vi "Aux CO2 Serial Write and Read.vi"(4 "error in":errorcluster, 5 "Action":T2, 6 "string to write":string, 7 "Serial Port":T1={"termination char"=10, "End read on termination character?"=TRUE, "Enabled?"=FALSE, "VISA resource name"="COM7", "baud rate"=9600, "data bits"=8, "parity"=enum."None", "stop bits"=10, "flow control"=0, "timeout (ms)"=10000, "Input buffer size"=4096, "End write on termination character?"=FALSE, "XON Char"=17, "XOFF Char"=19} {"XOFF Char" format="%.0x"; "XON Char" format="%.0x"; "flow control" items=["None"=0, "XON/XOFF"=1, "RTS/CTS"=2, "DTR/DSR"=4]; "stop bits" items=["1.0"=10, "1.5"=15, "2.0"=20]; "baud rate" items=["1.0"=10, "1.5"=15, "2.0"=20]; "termination char" format="%.0x"}) -> (0 "error IO":errorcluster, 1 "bytes read":i16=5, 2 "read string":string="\n", 3 "Serial Port Out":T1={"termination char"=10, "End read on termination character?"=TRUE, "Enabled?"=TRUE, "VISA resource name"="COM1", "baud rate"=9600, "data bits"=8, "parity"=enum."None", "stop bits"=10, "flow control"=0, "timeout (ms)"=10000, "Input buffer size"=4096, "End write on termination character?"=FALSE, "XON Char"=17, "XOFF Char"=19} {"XOFF Char" format="%.0x"; "XON Char" format="%.0x"; "flow control" items=["None"=0, "XON/XOFF"=1, "RTS/CTS"=2, "DTR/DSR"=4]; "stop bits" items=["1.0"=10, "1.5"=15, "2.0"=20]; "baud rate" items=["1.0"=10, "1.5"=15, "2.0"=20]; "termination char" format="%.0x"})   [LabVIEW 2016]
doc: "The Advanced Serial Read and Write example performs a Serial Port Read, a Serial Port Write, or a combination of these actions while setting some advanced serial features like buffer size, termination characters, and XON/XOFF flow control. The user selects the actions (read or write) on the front panel. If both are selected, the VI will write the data first, read the data and then close the VISA session that is opened to the port. \n\nThe parameters set for the serial port must match the parameters of the connected instrument or device. In this example, the bytes to read parameter specifies the number of bytes that the serial port reads. If there were more bytes at the port than the number specified in bytes to read, those bytes would not be read. Also, if you specify to read more bytes than the number of bytes actually read, you might receive a timeout error message.\n\nINSTRUCTIONS:\n1) Select the serial resource and configuration parameters (baud rate, data bits, parity, stop bits, flow control).\n2) Termination character can be enabled and set. Also, set the required input buffer size prior to running the example.\n3) Select the operations to be performed. \n4) Connect the serial port to your device. If no device is available, perform a loopback test by doing one of the following. Short pins 2 and 3 on a RS-232 cable or short pin 4 to pin 8 and pin 5 to pin 9 on a RS-485/422 cable. \n5) Run the VI to see the data read. (The \"read string\" will match the \"string to write\" if a loopback test was performed.)\n\nThis example exposes several advanced features that you may need for your application. Not all applications need all the features shown in this example. The input buffer size is likely an important setting that you want to control in your application. This example expands upon the flow control option for XON and XOFF, allowing the user to choose those control characters. The timeout parameter has been brought to the front panel so a user can specify the time period the VISA Read will wait for the number of bytes to read before timing out. Also, the user has several controls for the termination character, which is discussed later.\n\nNote that you can press the write and read buttons and change the bytes to read parameters on the fly, while the example is running. However, you must stop the example to change the other configuration parameters after the example has started running, and then run again.\n\nSet the I/O buffer size slightly higher the amount of data you expect to receive. This is very important for applications that don't use flow control, as you may lose characters if the receive buffer overflows.\n\nSetting the timeout period ensures that the operation returns with a timeout error if the operation cannot be performed in the specified time period. \n\nSome devices require a termination character in order to identify the end of command strings. Some devices send a termination character to signify the end of data to be read. \n\nThis example shows how you can end the Read operation once a termination character is detected in the buffer and/or append a termination character at the end of the Write data. To enable the Read to end on a termination character, use the VISA Configure Serial Port or use the VISA Properties Serial End Mode for Reads, Termination Character Enable, and Termination Character. To end the Write with a termination character, use the VISA Properties Serial End Mode for Writes, the Send End Enable, and Termination Character. In this example, the same termination character is used for both the Read and the Write. You can specify two different characters for your application, if desired.\n\nYour application may require specific characters for the XON/XOFF Flow Control. You can specify these characters with the VISA Properties Flow Control XOFF Character and Flow Control XON Character. Note that if the standard XON and XOFF characters are used, then decimal 17 and 19 are unavailable for data values. Remember that using flow control and setting an adequate buffer size allow you to prevent buffer overflows."
uses:
  Controls/Serial Visa Control.ctl
  Controls/SerialPortControl.ctl
  <vilib>/Instr/_visa.llb/VISA Configure Serial Port (Instr).vi
panel:
  # "Select the serial resource and the operations to be performed.  If all are selected, the VI will write the data first, read data and then close the VISA session that is opened to the port.  This VI will wait until the specified number of bytes is received at the port until the timeout period is met.  Only the specified number of bytes will be read unless the read ends on a termination character.  The termination character can be enabled and set.  Also, set the required input buffer size prior to running the example.\nNote: The example loops until the STOP button is pressed."
  # "For additional information select File >> VI Properties >> Documentation"
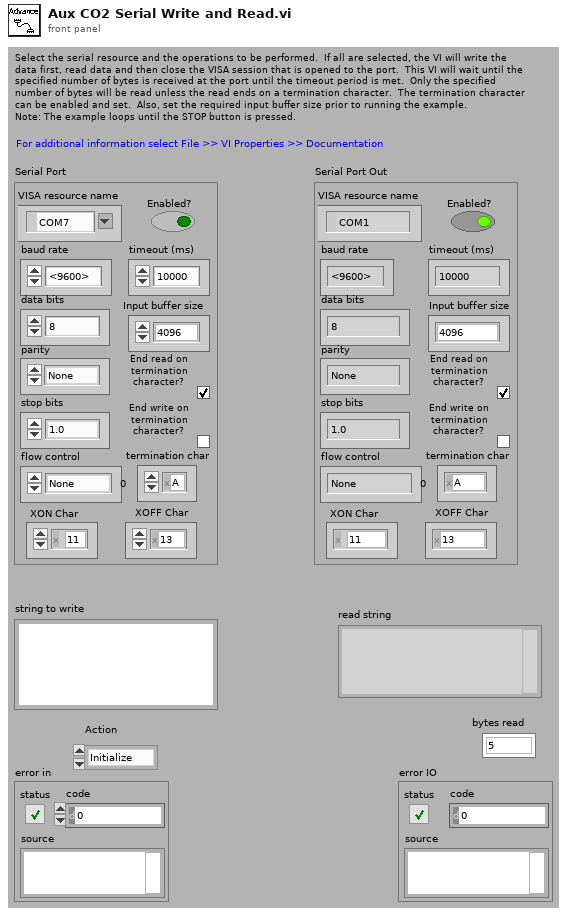
[diagram p1: front panel]
types:
  T1 = typedef "Serial Visa Control.ctl" = cluster{"termination char":u8, "End read on termination character?":bool, "Enabled?":bool, "VISA resource name":refnum<visa-resource-name>, "baud rate":u32, "data bits":u16, "parity":enum16{"None", "Odd", "Even", "Mark", "Space"}, "stop bits":u16, "flow control":u16, "timeout (ms)":u32, "Input buffer size":u32, "End write on termination character?":bool, "XON Char":u8, "XOFF Char":u8}
  T2 = typedef "SerialPortControl.ctl" = enum16{"Initialize", "Write Data", "Read Data", "Close Port"}
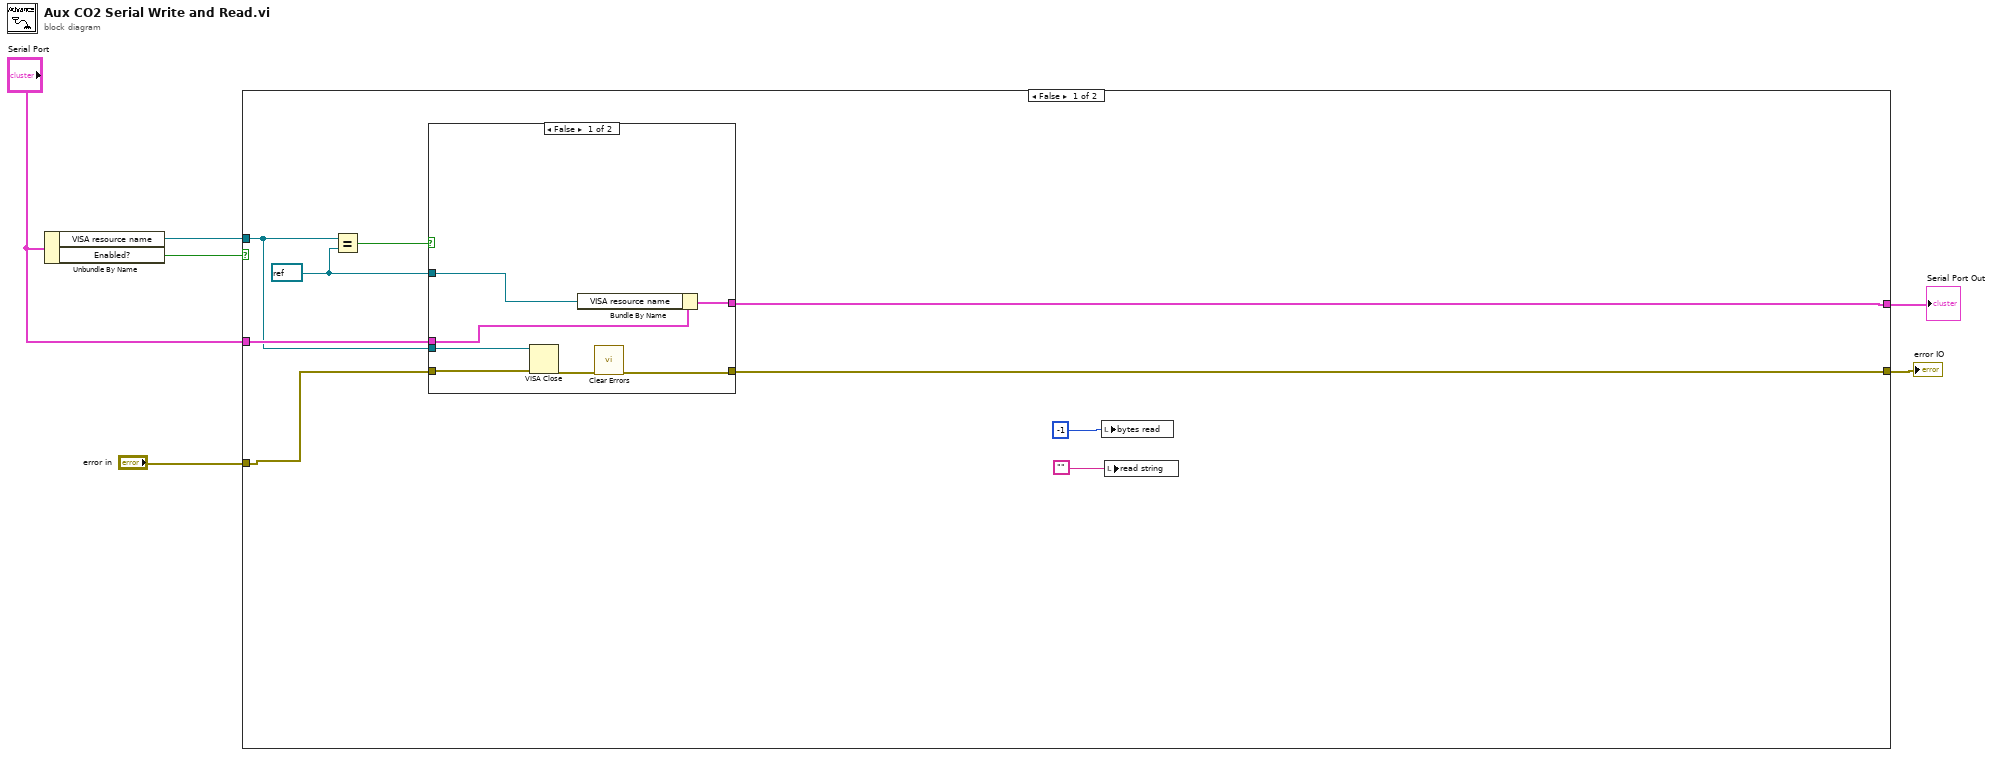
[diagram p0: block diagram]
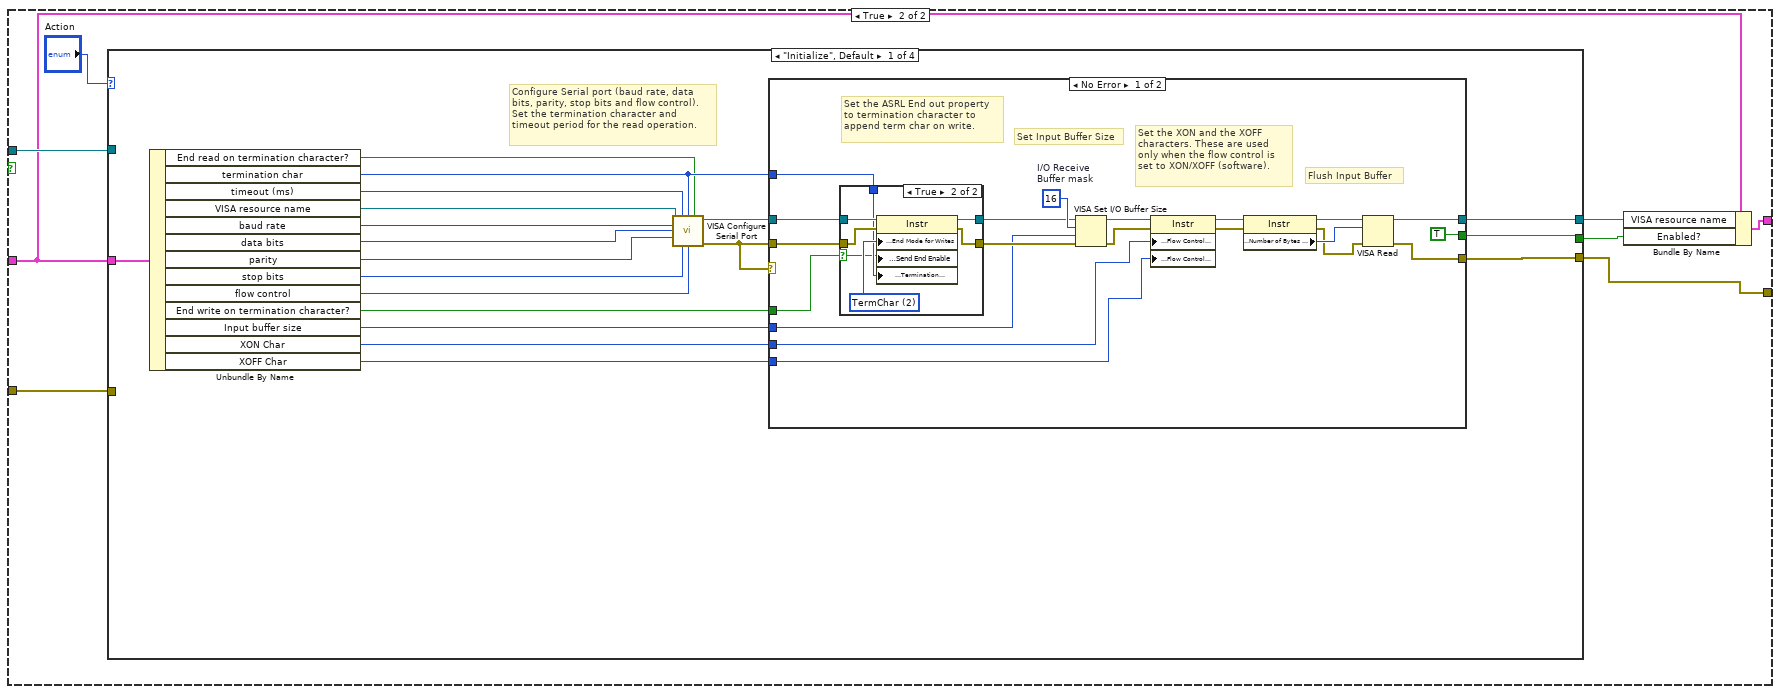
[diagram p3: hidden frame]
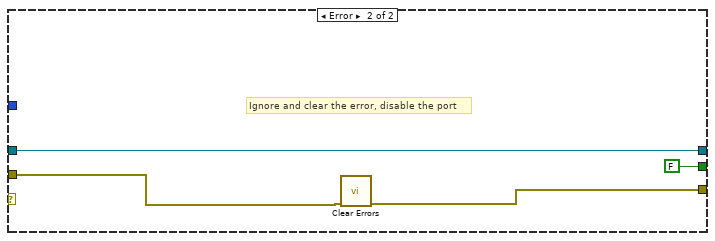
[diagram p5: hidden frame]
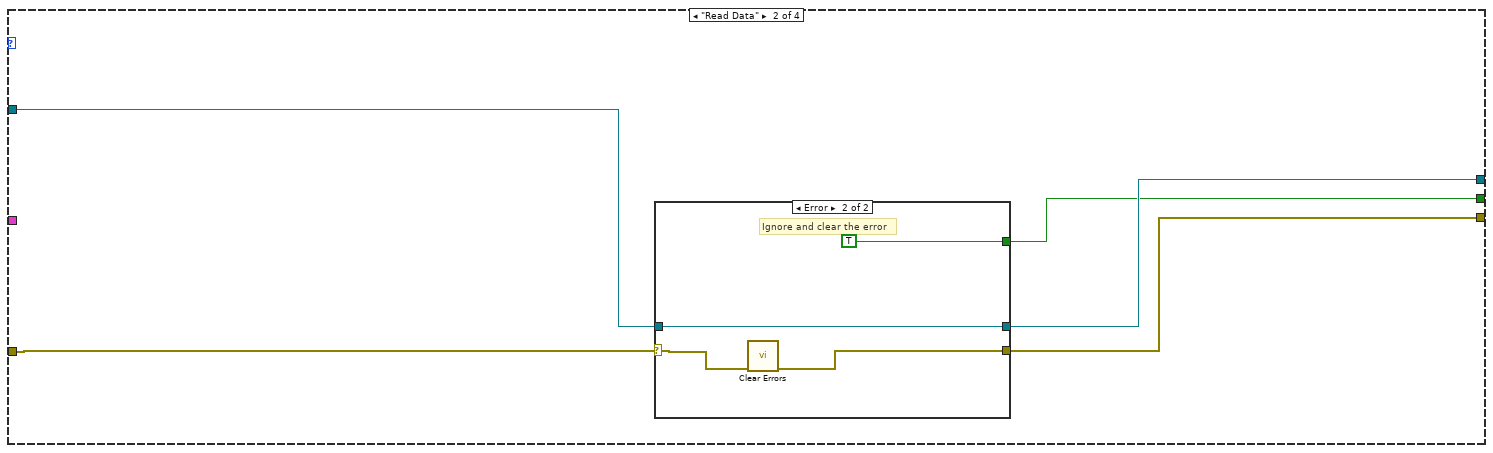
[diagram p6: hidden frame]
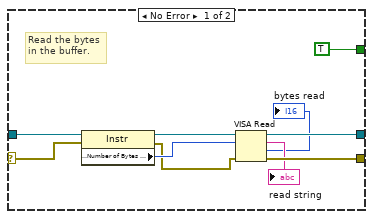
[diagram p7: hidden frame]
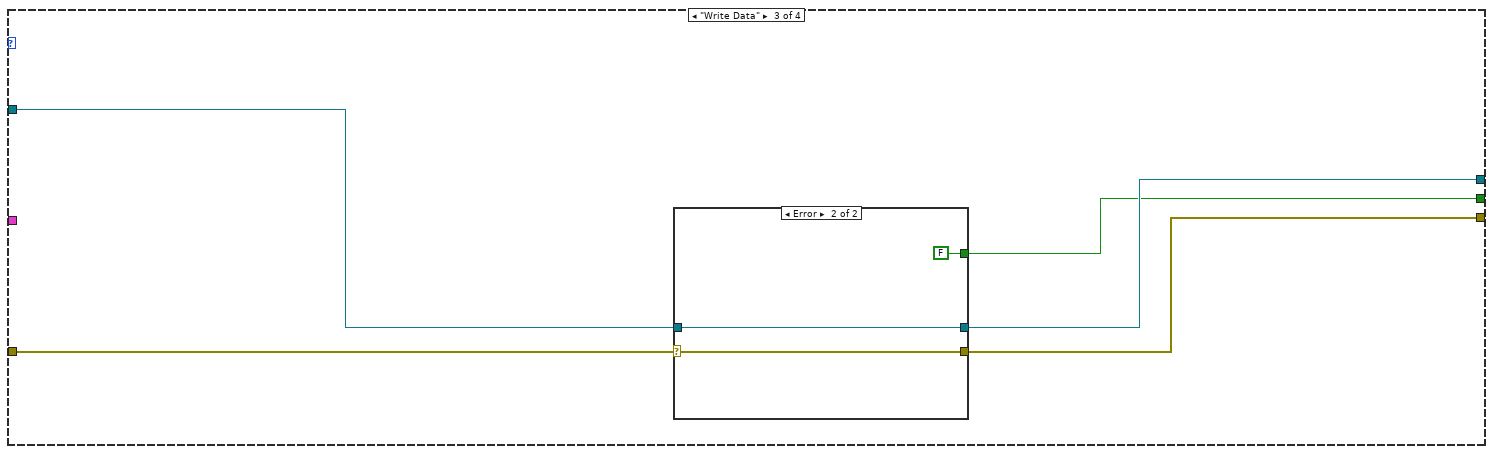
[diagram p8: hidden frame]
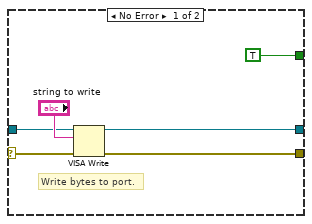
[diagram p9: hidden frame]
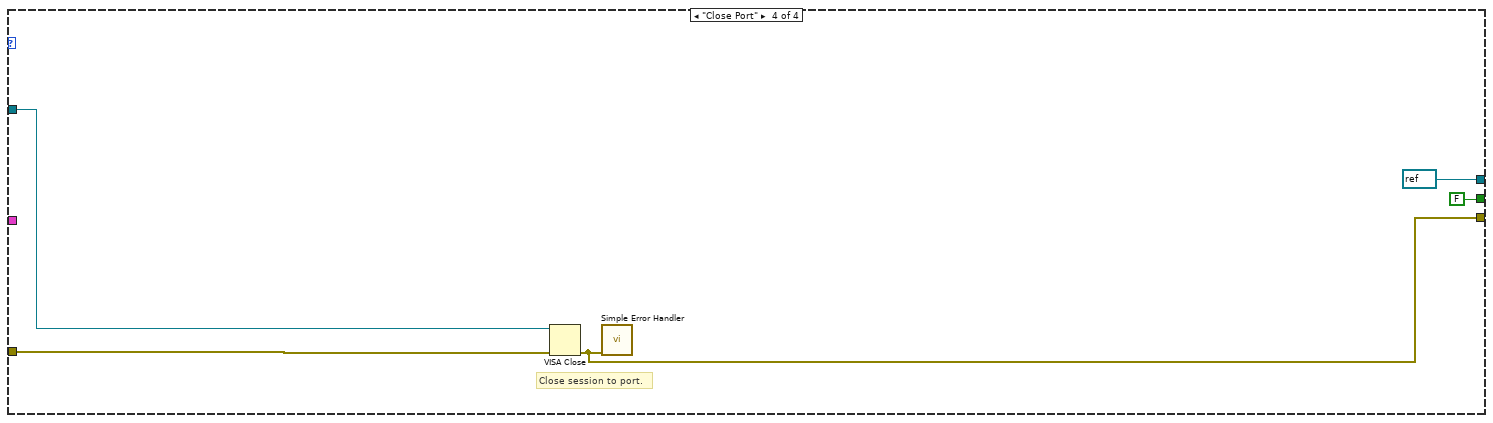
[diagram p10: hidden frame]
diagram:
  n1 = Unbundle By Name("Serial Port") -> ("VISA resource name"=w5:refnum<visa-resource-name>, "Enabled?"=w2:bool)
  n2 = case shown="False" w2 {
    tunnel: "error in" -> [w12 w31]
    tunnel: w5 -> [w7 w30]
    tunnel: "Serial Port" -> [w10 w26]
    tunnel: [w9 w28] -> w3
    tunnel: [w11 w27] -> w1
    frame False {
      w8 = refnum<visa-resource-name> refnum ("VISA resource name")
      n3 = Equal?(x=w7, y=w8) -> (x = y?=w13:bool)
      n4 = case shown="False" w13 {
        tunnel: w12 -> [w21 w24]
        tunnel: [w20 w24] -> w11
        tunnel: w8 -> [w17 _]
        tunnel: w10 -> [w18 w23]
        tunnel: [w19 w23] -> w9
        tunnel: w7 -> [w16 _]
        frame False {
          n5 = VISA Close(VISA resource name=w16, error in (no error)=w21) -> (error out=w22:errorcluster)
          n6 = Bundle By Name(cluster=w18, "VISA resource name"=w17) -> (w19:T1)
          n7 = call <vilib>:"Clear Errors.vi"("error in (no error)"=w22) -> ("error out"=w20:errorcluster)  [unwired: 5 in, 1 out]
        }
        frame True {
        }
      }
      n8 = local write "bytes read"(-1) -> ()
      n9 = local write "read string"("") -> ()
    }
    frame True {
      n10 = case shown="\"Initialize\", Default" "Action" {
        tunnel: [w51 w88 w108 w120] -> w27
        tunnel: [w49 w89 w107 refnum<visa-resource-name> refnum ("VISA resource name")] -> w29
        tunnel: w30 -> [_ w87 w106 w122]
        tunnel: w31 -> [_ w86 w105 w121]
        tunnel: w26 -> [w35 _ _ _]
        tunnel: [w33 w85 w104 FALSE] -> w25
        frame "Initialize", Default {
          # "Configure Serial port (baud rate, data\nbits, parity, stop bits and flow control).\nSet the termination character and\ntimeout period for the read operation."
          n11 = Unbundle By Name(w35) -> ("End read on termination character?"=w40:bool, "termination char"=w41:u8, "timeout (ms)"=w42:u32, "VISA resource name"=w48:refnum<visa-resource-name>, "baud rate"=w47:u32, "data bits"=w46:u16, "parity"=w45:enum16{"None", "Odd", "Even", "Mark", "Space"}, "stop bits"=w44:u16, "flow control"=w43:u16, "End write on termination character?"=w39:bool, "Input buffer size"=w38:u32, "XON Char"=w37:u8, "XOFF Char"=w36:u8)
          n12 = call-poly "VISA Configure Serial Port"("VISA resource name"=w48, "timeout (10sec)"=w42, "termination char\n(0xA = '\\n' = LF)"=w41, "Enable Termination\nChar (T)"=w40, "baud rate (9600)"=w47, "data bits (8)"=w46, "parity (0:none)"=w45, "stop bits (10: 1 bit)"=w44, "flow control (0:none)"=w43) -> ("VISA resource name out"=w50:refnum<visa-resource-name>, "error out"=w34:errorcluster)  [unwired: 5 in]
          n13 = case shown="No Error" w34 {
            tunnel: [w53 w82] -> w51
            tunnel: w34 -> [w68 w83]
            tunnel: w50 -> [w65 w84]
            tunnel: [w52 w84] -> w49
            tunnel: w41 -> [w64 _]
            tunnel: w39 -> [w63 _]
            tunnel: w38 -> [w62 _]
            tunnel: w37 -> [w61 _]
            tunnel: w36 -> [w60 _]
            tunnel: [TRUE FALSE] -> w33
            frame No Error {
              w71 = u16 16  # I/O Receive Buffer mask
              # "Flush Input Buffer"
              # "Set the XON and the XOFF\ncharacters. These are used\nonly when the flow control is\nset to XON/XOFF (software)."
              # "Set Input Buffer Size"
              # "Set the ASRL End out property\nto termination character to\nappend term char on write."
              n14 = case shown="True" w63 {
                selector: w63 -> [_ w74]
                tunnel: w65 -> [w72 w80]
                tunnel: w68 -> [w73 w79]
                tunnel: [w72 w78] -> w66
                tunnel: [w73 w77] -> w67
                tunnel: w64 -> [_ w75]
                frame False {
                }
                frame True {
                  w76 = u16 2 items=["None", "LastBit", "TermChar", "Break"] ("Serial Settings:Serial End Mode for Writes")
                  n15 = property class="Instr"(reference=w80, error in=w79, "Serial Settings:End Mode for Writes"=w76, "Message Based Settings:Send End Enable"=w74, "Message Based Settings:Termination Character"=w75) -> (reference out=w78:refnum<visa-resource-name>, error out=w77:errorcluster)
                }
              }
              n16 = VISA Set I/O Buffer Size(VISA resource name=w66, mask (16)=w71, size (4096)=w62, error in (no error)=w67) -> (VISA resource name out=w70:refnum<visa-resource-name>, error out=w69:errorcluster)
              n17 = property class="Instr"(reference=w70, error in=w69, "Serial Settings:Flow Control XON Character"=w61, "Serial Settings:Flow Control XOFF Character"=w60) -> (reference out=w55:refnum<visa-resource-name>, error out=w54:errorcluster)
              n18 = property class="Instr"(reference=w55, error in=w54) -> (reference out=w58:refnum<visa-resource-name>, error out=w56:errorcluster, "Serial Settings:Number of Bytes at Serial Port"=w57:u32)
              n19 = VISA Read(VISA resource name=w58, byte count=w57, error in (no error)=w56) -> (VISA resource name out=w52:refnum<visa-resource-name>, error out=w53:errorcluster)  [unwired: 2 out]
            }
            frame Error {
              # "Ignore and clear the error, disable the port"
              n20 = call <vilib>:"Clear Errors.vi"("error in (no error)"=w83) -> ("error out"=w82:errorcluster)  [unwired: 5 in, 1 out]
            }
          }
        }
        frame "Read Data" {
          n21 = case "Read bytes from port." shown="Error" w86 {
            selector: w86 -> [w90 w101]
            tunnel: [w98 w102] -> w88
            tunnel: [w99 w103] -> w89
            tunnel: w87 -> [w93 w103]
            tunnel: [TRUE TRUE] -> w85
            frame No Error {
              # "Read the bytes\nin the buffer."
              n22 = property class="Instr"(reference=w93, error in=w90) -> (reference out=w94:refnum<visa-resource-name>, error out=w91:errorcluster, "Serial Settings:Number of Bytes at Serial Port"=w92:u32)
              n23 = VISA Read(VISA resource name=w94, byte count=w92, error in (no error)=w91) -> (VISA resource name out=w99:refnum<visa-resource-name>, read buffer=→"read string":string, return count=→"bytes read":u32, error out=w98:errorcluster)
            }
            frame Error {
              # "Ignore and clear the error"
              # "Error occurred \nreading Bytes at \nSerial Port"
              n24 = call <vilib>:"Clear Errors.vi"("error in (no error)"=w101) -> ("error out"=w102:errorcluster)  [unwired: 5 in, 1 out]
            }
          }
        }
        frame "Write Data" {
          n25 = case shown="Error" w105 {
            selector: w105 -> [w110 w117]
            tunnel: [w114 w116] -> w107
            tunnel: [w113 w117] -> w108
            tunnel: w106 -> [w111 w116]
            tunnel: [TRUE FALSE] -> w104
            frame No Error {
              # "Write bytes to port."
              n26 = VISA Write(VISA resource name=w111, write buffer="string to write", error in (no error)=w110) -> (VISA resource name out=w114:refnum<visa-resource-name>, error out=w113:errorcluster)  [unwired: 1 out]
            }
            frame Error {
            }
          }
        }
        frame "Close Port" {
          # "Close session to port."
          n27 = VISA Close(VISA resource name=w122, error in (no error)=w121) -> (error out=w120:errorcluster)
          n28 = call <vilib>:"Simple Error Handler.vi"("error in (no error)"=w120) -> ()  [unwired: 4 in, 5 out]
        }
      }
      n29 = Bundle By Name(cluster=w26, "VISA resource name"=w29, "Enabled?"=w25) -> (w28:T1)
    }
  }
  "Serial Port Out" <- w3
  "error IO" <- w1
